vi "Configure RemIO Module Core.vi"(8 "error in (no error)":errorcluster, 9 "module slot index":u8=1, 10 "Slave Ref In":refnum<k21>, 11 "11115 in":refnum<class "11115.lvclass">) -> (0 "error out":errorcluster, 1 "negative confirmation":T1 {"additional error code" format="%.0x"; "error code" format="%.0x"}, 2 "Slave Ref Out":refnum<k21>, 3 "11115 out":refnum<class "11115.lvclass">, 5 "SDO abort code":u32 format="%.0x")   [LabVIEW 2017, in "Modules.lvlib" / "11115.lvclass"]
uses:
  11115.lvclass
  <vilib>/indcomecat/Remote IO/typedefs/negative confirmation.ctl
  11115.lvclass/11115.ctl
  RemIO Module/RemIO Module.lvclass
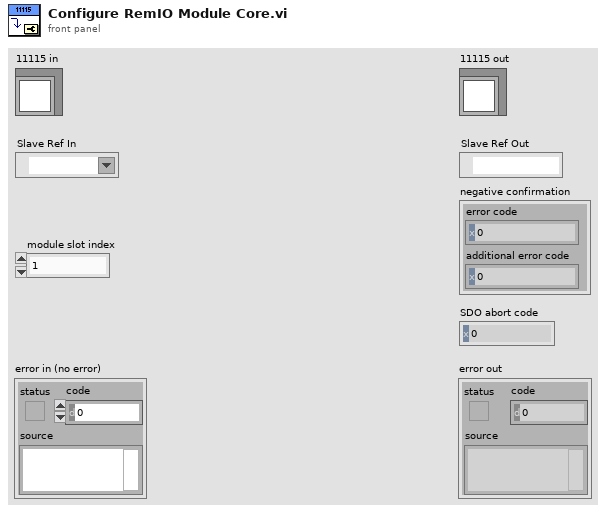
[diagram p1: front panel]
types:
  T1 = typedef "negative confirmation.ctl" = cluster{"error code":u16, "additional error code":u16}
  T2 = typedef "NI ECAT Remote IO.lvlib/channel number REM-11115.ctl" = u8
  T3 = typedef "NI ECAT Remote IO.lvlib/output range REM-11115.ctl" = u8
  T4 = cluster{"channel number":T2, "output range":T3}[]
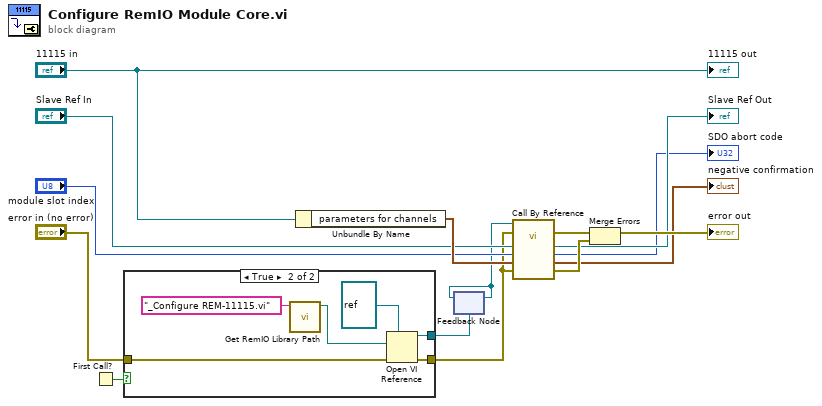
[diagram p0: block diagram]
diagram:
  n1 = First Call?() -> (First Call?: T/F=w5:bool)
  n2 = case shown="True" w5 {
    tunnel: [_ w20] -> w4
    tunnel: [w16 w19] -> w2
    tunnel: "error in (no error)" -> [w16 w18]
    frame False {
    }
    frame True {
      n3 = call "Get RemIO Library Path.vi"("name or relative path"="_Configure REM-11115.vi") -> ("appended path"=w21:path)  [unwired: 10 in]
      n4 = Open VI Reference(type specifier VI Refnum (for type only)=refnum<vi> refnum, vi path=w21, error in (no error)=w18) -> (vi reference=w20:refnum<vi>, error out=w19:errorcluster)  [unwired: 3 in]
    }
  }
  n5 = Unbundle By Name("11115 in") -> ("parameters for channels"=w11:T4)
  n6 = feedback #1(w4) -> (w1:refnum<vi>)
  n7 = feedback-in #1(w1) -> ()
  n8 = call-by-ref "?"(reference=w1, error in=w2, 8:"error in (no error)"=w2, "parameters for channels"=w11, "module slot index"="module slot index", "slave reference in"="Slave Ref In") -> (error out=w13:errorcluster, 0:"error out"=w14:errorcluster, "negative confirmation"=→"negative confirmation":T1, "SDO abort code"=→"SDO abort code":u32, "slave reference out"=→"Slave Ref Out":refnum<k21>)  [unwired: 4 in, 1 out]
  n9 = Merge Errors(w13, w14) -> (→"error out":errorcluster)
  "11115 out" <- "11115 in"
